vi "InitializeDVR.vi"(8 "error in (no error)":errorcluster, 11 "MicronGRPCClient in":refnum<class "MicronGRPCClient.lvclass">) -> (0 "error out":errorcluster, 3 "MicronGRPCClient out":refnum<class "MicronGRPCClient.lvclass">)   [LabVIEW 2019, in "MicronGRPCClient.lvclass"]
uses:
  MicronGRPCClient.lvclass
  MicronGRPCClient.lvclass/MicronGRPCClient.ctl
  Typedefs/InternalCluster.ctl
  Base/Client/Typedefs/ServiceDetails.ctl
  Typedefs/gRPCDetails.ctl
  <vilib>/gRPC/LabVIEW gRPC Library/Shared/grpcId.ctl
  Base/Client/MicronClient.lvclass
  <vilib>/gRPC/LabVIEW gRPC Library/grpc-lvsupport-release.lvlib
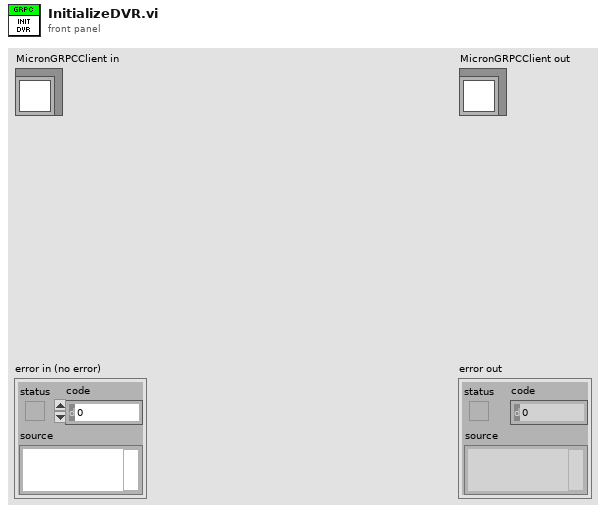
[diagram p1: front panel]
types:
  T1 = typedef "MicronGRPCClient.lvclass/InternalCluster.ctl" = cluster{"ServiceDetails":T2, "gRPCDetails":T3}
  T2 = typedef "MicronClient.lvclass/ServiceDetails.ctl" = cluster{"MicronPath":path, "Network":string, "ServiceID":string, "Port":i32, "FullyQualifiedName":string, "UI":string, "Args":string, "Mode":string, "AutoRestartOnError?":bool, "Simulate?":bool}
  T3 = typedef "MicronGRPCClient.lvclass/gRPCDetails.ctl" = cluster{"ConnectionString":string, "ID":T4, "PackageName":string, "ServiceName":string}
  T4 = typedef "grpc-lvsupport-release.lvlib/grpcId.ctl" = u64
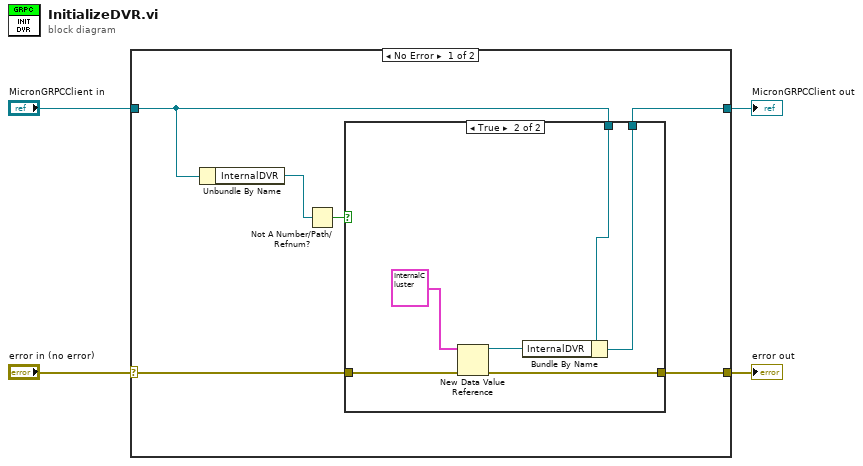
[diagram p0: block diagram]
diagram:
  n1 = case shown="No Error" "error in (no error)" {
    selector: "error in (no error)" -> [w9 w20]
    tunnel: [w10 w20] -> w3
    tunnel: [w8 w19] -> w1
    tunnel: "MicronGRPCClient in" -> [w7 w19]
    frame No Error {
      n2 = Unbundle By Name(w7) -> ("InternalDVR"=w6:refnum<data-value>)
      n3 = Not A Number/Path/Refnum?(number/path/refnum=w6) -> (NaN/Path/Refnum?=w5:bool)
      n4 = case shown="True" w5 {
        tunnel: [w11 w18] -> w10
        tunnel: w9 -> [w11 w17]
        tunnel: [w12 w15] -> w8
        tunnel: w7 -> [w12 w13]
        frame False {
        }
        frame True {
          n5 = New Data Value Reference(data value=T1 {"ServiceDetails"={"MicronPath"=path "", "Network"="", "ServiceID"="", "Port"=0, "FullyQualifiedName"="", "UI"="", "Args"="", "Mode"="", "AutoRestartOnError?"=FALSE, "Simulate?"=FALSE}, "gRPCDetails"={"ConnectionString"="", "ID"=0, "PackageName"="", "ServiceName"=""}} ("gRPC"), error in=w17) -> (data value reference=w16:refnum<data-value>, error out=w18:errorcluster)
          n6 = Bundle By Name(cluster=w13, "InternalDVR"=w16) -> (w15:refnum<class "MicronGRPCClient.lvclass">)
        }
      }
    }
    frame Error {
    }
  }
  "error out" <- w3
  "MicronGRPCClient out" <- w1
